vi "Write String Configuration.vi"(8 "error in (no error)":errorcluster, 9 "Value":string, 10 "Name":string, 11 "database-configuration in":refnum<class "configuration-database.lvclass">) -> (0 "error out":errorcluster, 3 "database-configuration out":refnum<class "configuration-database.lvclass">)   [LabVIEW 2020, in "configuration-database.lvlib" / "configuration-database.lvclass"]
uses:
  configuration-database.lvclass
  configuration-database.lvclass/configuration-database.ctl
  c43f59e4-2e36-4b61-b898-6c01ce4671d9.vi
  <vilib>/Utility/error.llb/Error Cluster From Error Code.vi
  IConfigDBQueries/IConfigurationDatabaseQueries.lvclass
  externals/database-interface/IDatabase/IDatabase/IDatabase.lvclass
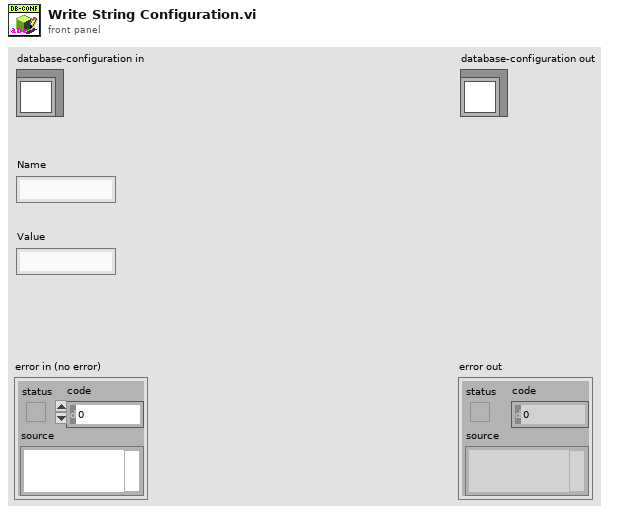
[diagram p1: front panel]
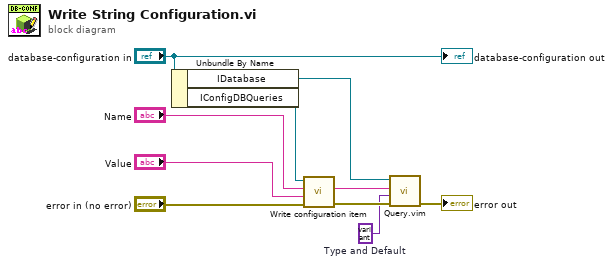
[diagram p0: block diagram]
diagram:
  w1 = variant  # Type and Default
  n1 = Unbundle By Name("database-configuration in") -> ("IDatabase"=w7:refnum<class "IDatabase.lvclass">, "IConfigDBQueries"=w8:refnum<class "IConfigurationDatabaseQueries.lvclass">)
  n2 = call-dynamic "Write configuration item.vi"("error in (no error)"="error in (no error)", "Value"="Value", "Name in"="Name", "IConfigDBQueries in"=w8) -> ("error out"=w9:errorcluster, "Query"=w10:string)  [unwired: 6 in]
  n3 = call "Query.vim"("error in (no error)"=w9, "Type and Default"=w1, "Query string"=w10, "IDatabase in"=w7) -> ("error out"=→"error out":errorcluster)  [unwired: 5 in, 2 out]
  "database-configuration out" <- "database-configuration in"
